vi "GitDiffCommits.vi"(6 "Old Hash (HEAD)":string="HEAD", 7 "New Hash":string, 8 "error in (no error)":errorcluster, 9 "File":path=path "", 11 "Git exec":string="git") -> (0 "error out":errorcluster, 1 "File out":path, 2 "Response":string, 3 "Git exec out":string="git", 4 "Differ":bool)   [LabVIEW 2013]
uses:
  GitCmd.vi
  <vilib>/Utility/error.llb/General Error Handler.vi
  GitUtils/PathtoDirPath.vi
  <vilib>/Platform/system.llb/System Exec.vi
  <vilib>/Utility/error.llb/Error Cluster From Error Code.vi
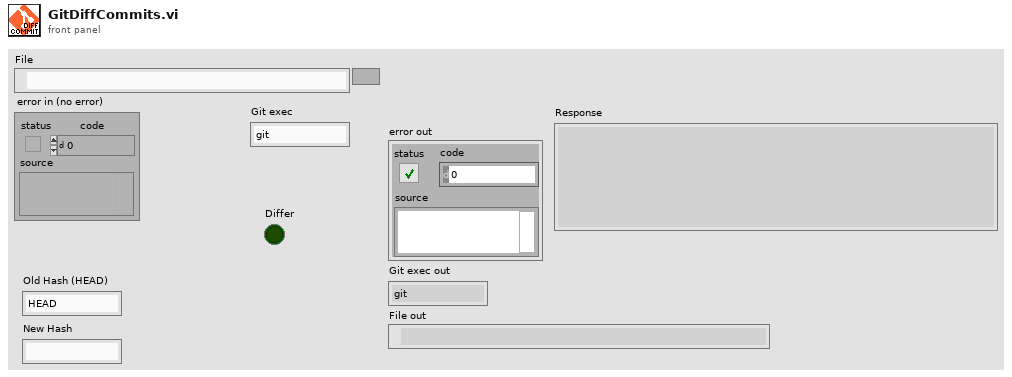
[diagram p1: front panel]
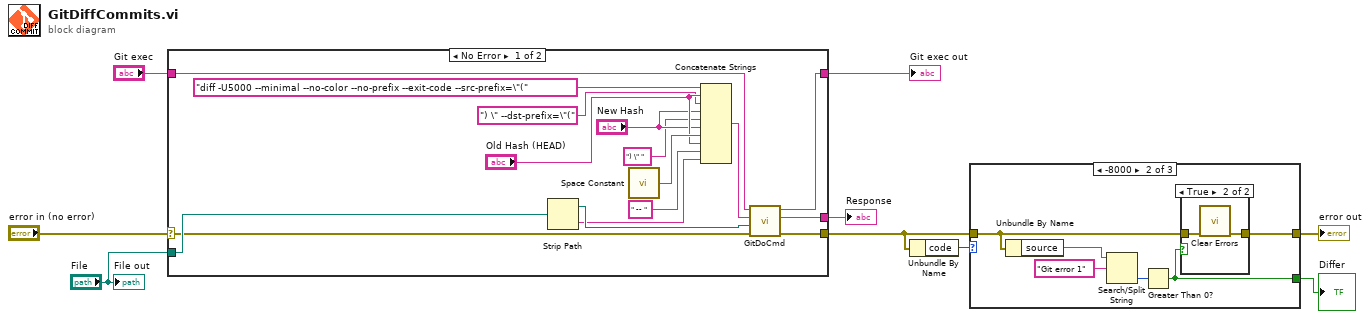
[diagram p0: block diagram]
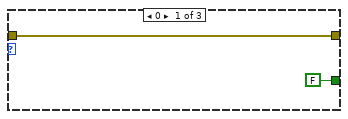
[diagram p2: hidden frame]
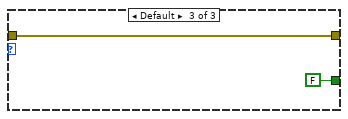
[diagram p4: hidden frame]
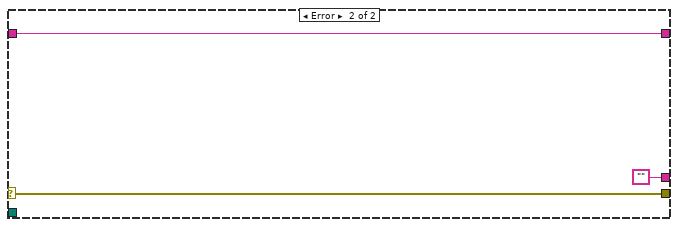
[diagram p5: hidden frame]
diagram:
  n1 = case shown="No Error" "error in (no error)" {
    selector: "error in (no error)" -> [w20 w27]
    tunnel: "Git exec" -> [w24 w26]
    tunnel: "File" -> [w25 _]
    tunnel: [w22 ""] -> w1
    tunnel: [w19 w27] -> w3
    tunnel: [w23 w26] -> w6
    frame No Error {
      n2 = Strip Path(path=w25) -> (stripped path=w21:path, name=w15:string)
      n3 = call <vilib>:"Space Constant.vi"() -> ("String"=w17:string)
      n4 = Concatenate Strings("diff -U5000 --minimal --no-color --no-prefix --exit-code --src-prefix=\"(" ("string"), "Old Hash (HEAD)", ") \" --dst-prefix=\"(" ("string"), "New Hash", ") \" " ("string"), "New Hash", w17, "Old Hash (HEAD)", " -- " ("string"), w15) -> (w14:string)
      n5 = call "GitDoCmd.vi"("error in (no error)"=w20, "Working Path"=w21, "Git command"=w14, "Git exec"=w24) -> ("error out"=w19:errorcluster, "Returned stdout"=w22:string, "Git exec out"=w23:string)  [unwired: 3 in, 1 out]
    }
    frame Error {
    }
  }
  "Response" <- w1
  "Git exec out" <- w6
  n6 = Unbundle By Name(w3) -> ("code"=w5:i32)
  n7 = case shown="-8000" w5 {
    tunnel: [w30 w32 w41] -> w4
    tunnel: w3 -> [w30 w33 w41]
    tunnel: [FALSE ("Differ") w31 FALSE ("Differ")] -> w2
    frame 0 {
    }
    frame -8000 {
      n8 = Unbundle By Name(w33) -> ("source"=w35:string)
      n9 = Search/Split String(string=w35, search string/char (-)="Git error 1") -> (offset of match=w36:i32)  [unwired: 1 in, 2 out]
      n10 = Greater Than 0?(x=w36) -> (x > 0?=w31:bool)
      n11 = case shown="True" w31 {
        tunnel: w33 -> [w37 w39]
        tunnel: [w37 w38] -> w32
        frame False {
        }
        frame True {
          n12 = call <vilib>:"Clear Errors.vi"("error in (no error)"=w39) -> ("error out"=w38:errorcluster)  [unwired: 6 in]
        }
      }
    }
    frame Default {
    }
  }
  "error out" <- w4
  "Differ" <- w2
  "File out" <- "File"
